vi "Send Notification.vi"(4 "Paras In 2":variant, 6 "Paras In":variant, 7 "Timeout":i32=-1, 8 "error in (no error)":errorcluster, 9 "Notification In":variant, 10 "Mail Strategy":refnum<class "Mail Strategy.lvclass">, 11 "Simple Map Notifier Controller in":refnum<class "Simple Map SEQ I64 Notifier Controller.lvclass">) -> (0 "error out":errorcluster, 3 "Simple Map Notifier Controller out":refnum<class "Simple Map SEQ I64 Notifier Controller.lvclass">)   [LabVIEW 2022 SP3, in "Simple Map SEQ I64 Notifier Controller.lvclass"]
uses:
  Simple Map SEQ I64 Notifier Controller.lvclass
  Ancestor Class/Messenger/Mail Strategy/Mail Strategy.lvclass
  Simple Map SEQ I64 Notifier Controller.lvclass/Simple Map SEQ I64 Notifier Controller.ctl
  Ancestor Class/Actor Assistant/Notifier/Notifier.lvclass
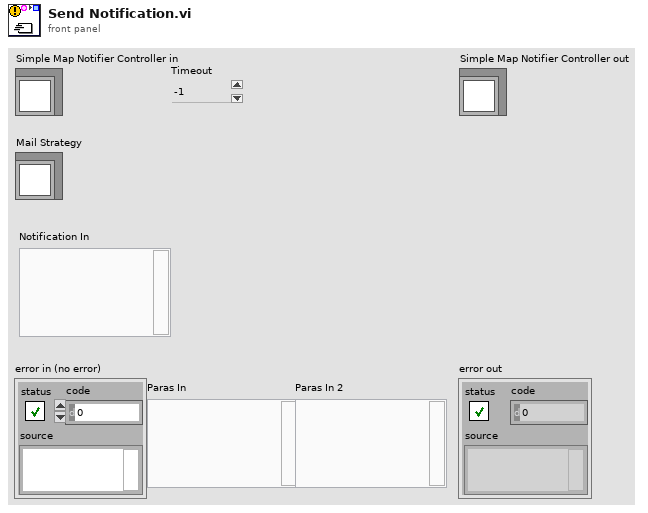
[diagram p1: front panel]
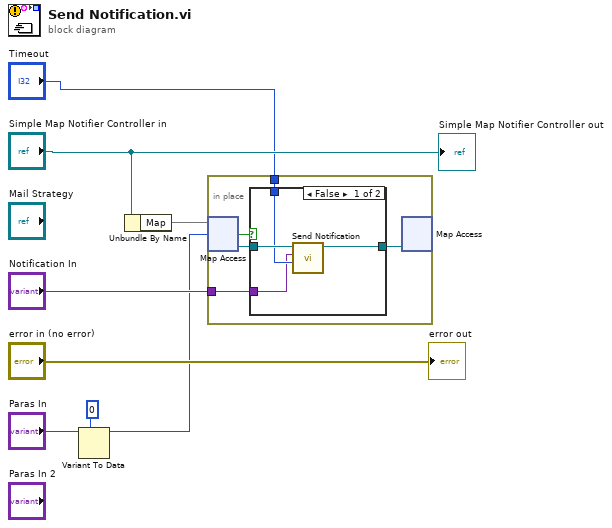
[diagram p0: block diagram]
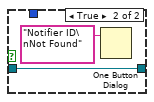
[diagram p2: hidden frame]
diagram:
  n1 = Variant To Data(type=i64 0, Variant="Paras In") -> (data=w1:i64)  [unwired: 1 in, 1 out]
  n2 = Unbundle By Name("Simple Map Notifier Controller in") -> ("Map"=w6:map{i64, refnum<class "Notifier.lvclass">})
  n3 = in-place {
    in-place-border: "Timeout" -> [w10]
    in-place-border: "Notification In" -> [w9]
    n4 = in-place-map #1(w6, w1) -> (w12:refnum<class "Notifier.lvclass">, w13:bool)  [unwired: 1 in]
    n5 = case shown="False" w13 {
      tunnel: w12 -> [w17 w18]
      tunnel: [w16 w18] -> w11
      tunnel: w10 -> [w15 _]
      tunnel: w9 -> [w14 _]
      frame False {
        n6 = call-dynamic "Send Notification.vi"("Timeout"=w15, "Notification"=w14, "Notifier in"=w17) -> ("Notifier out"=w16:refnum<class "Notifier.lvclass">)  [unwired: 6 in, 2 out]
      }
      frame True {
        n7 = One Button Dialog(message="Notifier ID\nNot Found") -> ()  [unwired: 1 in, 1 out]
      }
    }
    n8 = in-place-map #1(w11) -> ()  [unwired: 1 in, 3 out]
  }
  "error out" <- "error in (no error)"
  "Simple Map Notifier Controller out" <- "Simple Map Notifier Controller in"
